vi "Get_Ao_Array.vi"(0 "reference in":refnum<class "FPGA_Interface.lvclass">, 11 "error in (no error)":errorcluster) -> (4 "reference out":refnum<class "FPGA_Interface.lvclass">, 6 "AOs":dbl[](array[numeric]), 15 "error out":errorcluster)   [LabVIEW 2019, in "FPGA_Interface.lvclass"]
uses:
  FPGA_Interface.lvclass
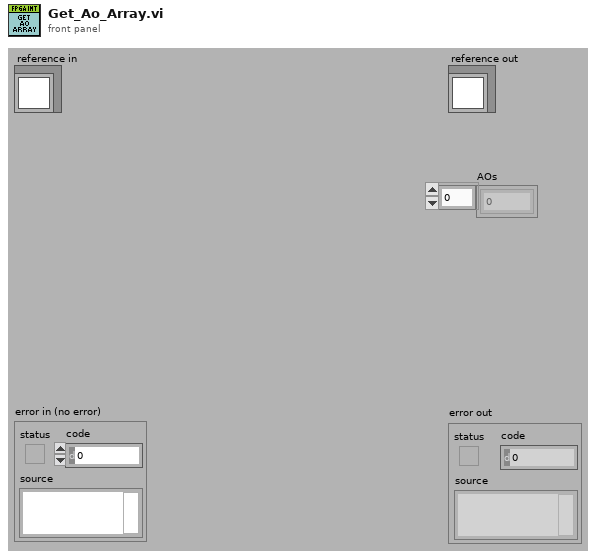
[diagram p1: front panel]
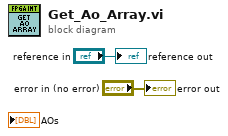
[diagram p0: block diagram]
diagram:
  "error out" <- "error in (no error)"
  "reference out" <- "reference in"
